vi "overlayfillcircle.vi"(0 "引用句柄输入":T1, 1 "数值":u8=25, 3 "Point1 (Pixels)":cluster{"X":sgl, "Y":sgl}, 5 "中心":cluster{"X":dbl, "Y":dbl}, 9 "偏移":cluster{"X":dbl, "Y":dbl}, 11 "错误输入（无错误）":errorcluster, 12 "分辨率":cluster{"X":sgl, "Y":sgl}={"X"=0.005, "Y"=0.005}, 14 "Point2 (Pixels)":cluster{"X":sgl, "Y":sgl}) -> (4 "引用句柄输出":T1, 10 "Point":cluster{"X":dbl, "Y":dbl}, 15 "错误输出":errorcluster)   [LabVIEW 2015]
uses:
  <vilib>/vision/Image Controls.llb/IMAQ Image.ctl
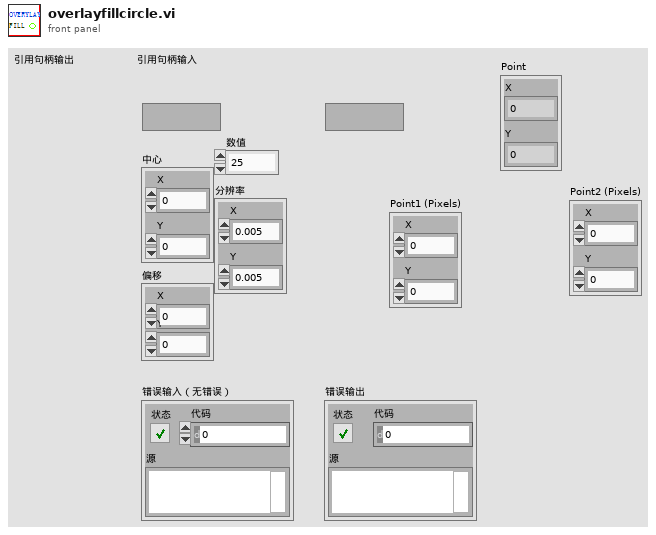
[diagram p1: front panel]
types:
  T1 = typedef "IMAQ Image.ctl" = refnum<image>
  T2 = cluster{"Left":i32, "Top":i32, "Right":i32, "Bottom":i32}
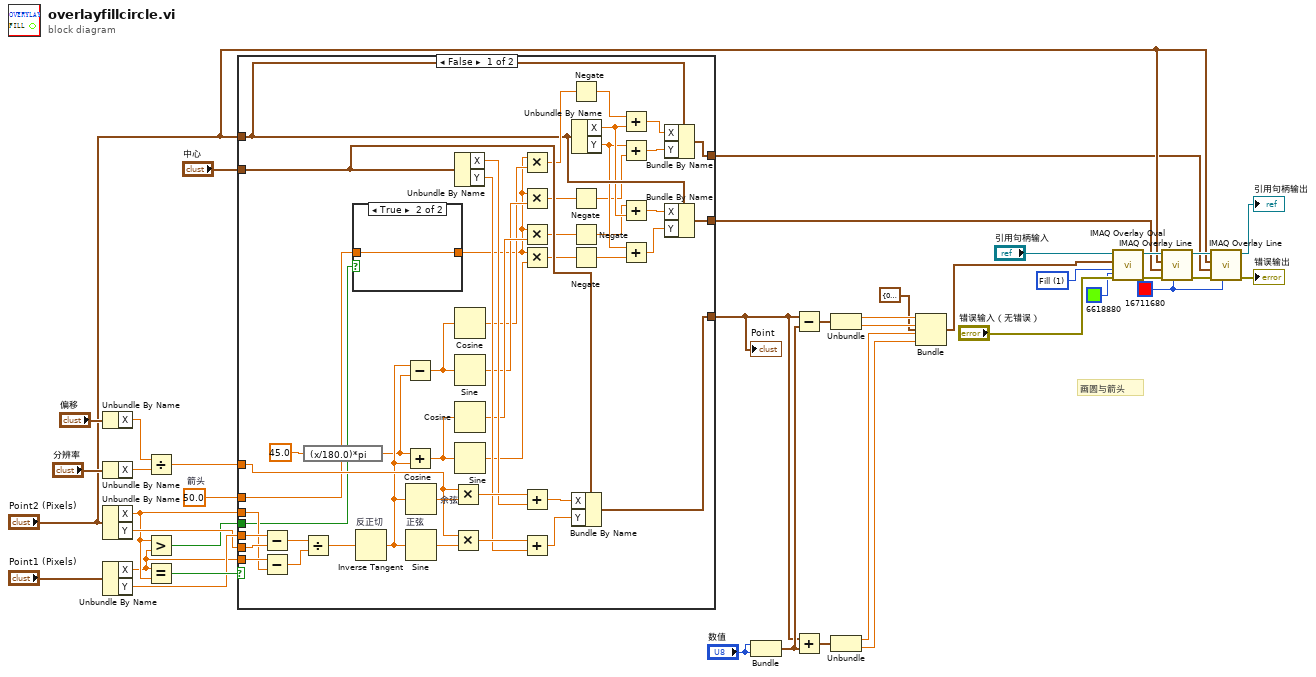
[diagram p0: block diagram]
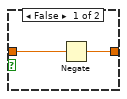
[diagram p2: hidden frame]
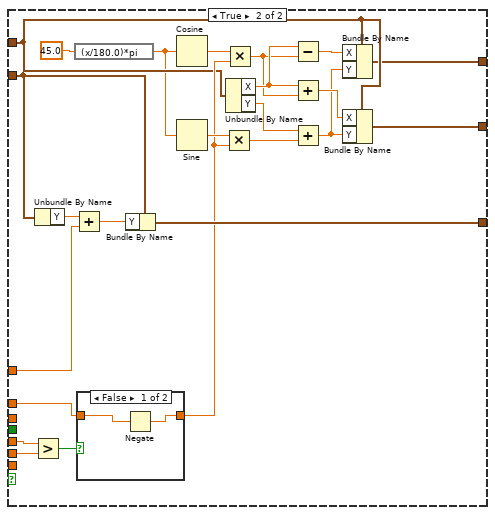
[diagram p3: hidden frame]
diagram:
  w1 = u32 16711680 ("Color")
  w5 = sgl 50.0  # 箭头
  w29 = u32 1 items=["Frame", "Fill"] ("Drawing Mode (Frame)")
  # "画圆与箭头"
  n1 = Unbundle By Name("偏移") -> ("X"=w22:dbl)
  n2 = Unbundle By Name("分辨率") -> ("X"=w20:sgl)
  n3 = Unbundle By Name("Point2 (Pixels)") -> ("X"=w8:sgl, "Y"=w16:sgl)
  n4 = Unbundle By Name("Point1 (Pixels)") -> ("X"=w7:sgl, "Y"=w17:sgl)
  n5 = Divide(x=w22, y=w20) -> (x/y=w18:dbl)
  n6 = Greater?(x=w8, y=w7) -> (0:w6:bool)
  n7 = Equal?(x=w7, y=w8) -> (x = y?=w24:bool)
  n8 = case shown="False" w24 {
    tunnel: "中心" -> [w77 w111]
    tunnel: w18 -> [w55 w113]
    tunnel: [w74 w112] -> w15
    tunnel: w17 -> [w86 w108]
    tunnel: w16 -> [w73 w107]
    tunnel: w7 -> [w46 _]
    tunnel: w8 -> [w45 _]
    tunnel: "Point2 (Pixels)" -> [w57 w98]
    tunnel: [w64 w99] -> w10
    tunnel: [w56 w97] -> w9
    tunnel: w6 -> [w44 _]
    tunnel: w5 -> [w40 w90]
    frame False {
      n9 = Subtract(x=w86, y=w73) -> (x-y=w85:sgl)
      n10 = Subtract(x=w46, y=w45) -> (x-y=w84:sgl)
      n11 = Divide(x=w85, y=w84) -> (x/y=w83:sgl)
      n12 = expression code="(x/180.0)*pi" ("degrees to radians")(45.0 ("Rotation")) -> (w41:dbl)
      n13 = case shown="True" w44 {
        tunnel: [w87 w89] -> w51
        tunnel: w40 -> [w88 w89]
        frame False {
          n14 = Negate(x=w88) -> (-x=w87:sgl)
        }
        frame True {
        }
      }
      n15 = Inverse Tangent "反正切"(1:w83) -> (0:w42:sgl)
      n16 = Subtract(x=w42, y=w41) -> (x-y=w63:dbl)
      n17 = Add(x=w41, y=w42) -> (x+y=w65:dbl)
      n18 = Cosine "余弦"(x=w42) -> (cos(x)=w72:sgl)
      n19 = Sine "正弦"(x=w42) -> (sin(x)=w82:sgl)
      n20 = Multiply(x=w55, y=w72) -> (x*y=w81:dbl)
      n21 = Multiply(x=w55, y=w82) -> (x*y=w79:dbl)
      n22 = Unbundle By Name(w77) -> ("X"=w80:dbl, "Y"=w78:dbl)
      n23 = Cosine(x=w63) -> (cos(x)=w58:dbl)
      n24 = Sine(x=w63) -> (sin(x)=w59:dbl)
      n25 = Cosine(x=w65) -> (cos(x)=w71:dbl)
      n26 = Sine(x=w65) -> (sin(x)=w70:dbl)
      n27 = Multiply(x=w51, y=w58) -> (x*y=w60:dbl)
      n28 = Multiply(x=w51, y=w59) -> (x*y=w61:dbl)
      n29 = Multiply(x=w51, y=w71) -> (x*y=w69:dbl)
      n30 = Multiply(x=w51, y=w70) -> (x*y=w68:dbl)
      n31 = Add(x=w81, y=w80) -> (x+y=w76:dbl)
      n32 = Add(x=w79, y=w78) -> (x+y=w75:dbl)
      n33 = Negate(x=w60) -> (-x=w47:dbl)
      n34 = Negate(x=w61) -> (-x=w48:dbl)
      n35 = Negate(x=w69) -> (-x=w49:dbl)
      n36 = Negate(x=w68) -> (-x=w50:dbl)
      n37 = Unbundle By Name(w57) -> ("X"=w54:sgl, "Y"=w53:sgl)
      n38 = Bundle By Name(cluster=w77, "X"=w76, "Y"=w75) -> (w74:cluster{"X":dbl, "Y":dbl})
      n39 = Add(x=w47, y=w54) -> (x+y=w62:dbl)
      n40 = Add(x=w53, y=w48) -> (x+y=w52:dbl)
      n41 = Add(x=w49, y=w54) -> (x+y=w66:dbl)
      n42 = Add(x=w53, y=w50) -> (x+y=w67:dbl)
      n43 = Bundle By Name(cluster=w57, "X"=w62, "Y"=w52) -> (w56:cluster{"X":sgl, "Y":sgl})
      n44 = Bundle By Name(cluster=w57, "X"=w66, "Y"=w67) -> (w64:cluster{"X":sgl, "Y":sgl})
    }
    frame True {
      n45 = Greater?(x=w108, y=w107) -> (0:w106:bool)
      n46 = Unbundle By Name(w111) -> ("Y"=w109:dbl)
      n47 = Add(x=w109, y=w113) -> (x+y=w110:dbl)
      n48 = expression code="(x/180.0)*pi" ("degrees to radians")(45.0 ("Rotation")) -> (w92:dbl)
      n49 = case shown="False" w106 {
        tunnel: [w114 w116] -> w103
        tunnel: w90 -> [w115 w116]
        frame False {
          n50 = Negate(x=w115) -> (-x=w114:sgl)
        }
        frame True {
        }
      }
      n51 = Bundle By Name(cluster=w111, "Y"=w110) -> (w112:cluster{"X":dbl, "Y":dbl})
      n52 = Cosine(x=w92) -> (cos(x)=w105:dbl)
      n53 = Sine(x=w92) -> (sin(x)=w104:dbl)
      n54 = Multiply(x=w104, y=w103) -> (x*y=w101:dbl)
      n55 = Multiply(x=w105, y=w103) -> (x*y=w95:dbl)
      n56 = Unbundle By Name(w98) -> ("X"=w96:sgl, "Y"=w102:sgl)
      n57 = Subtract(x=w96, y=w95) -> (x-y=w94:dbl)
      n58 = Add(x=w96, y=w95) -> (x+y=w100:dbl)
      n59 = Add(x=w102, y=w101) -> (x+y=w93:dbl)
      n60 = Bundle By Name(cluster=w98, "X"=w94, "Y"=w93) -> (w97:cluster{"X":sgl, "Y":sgl})
      n61 = Bundle By Name(cluster=w98, "X"=w100, "Y"=w93) -> (w99:cluster{"X":sgl, "Y":sgl})
    }
  }
  "Point" <- w15
  n62 = Bundle("数值"="数值", "数值"="数值") -> (w26:cluster{"数值":u8, "数值":u8})  [unwired: 1 in]
  n63 = Subtract(x=w15, y=w26) -> (x-y=w31:cluster{dbl, dbl})
  n64 = Add(x=w15, y=w26) -> (x+y=w34:cluster{dbl, dbl})
  n65 = Unbundle(w31) -> (w32:dbl, w33:dbl)
  n66 = Unbundle(w34) -> (w35:dbl, w36:dbl)
  n67 = Bundle(cluster=T2 {"Left"=0, "Top"=0, "Right"=0, "Bottom"=0} ("Bounding Rectangle"), "Left"=w32, "Top"=w33, "Right"=w35, "Bottom"=w36) -> (w37:T2)
  n68 = call "IMAQ Overlay Oval"("Color"=u32 6618880, "error in (no error)"="错误输入（无错误）", "Drawing Mode (Frame)"=w29, "Bounding Rectangle"=w37, "Image"="引用句柄输入") -> ("error out"=w4:errorcluster, "Image Out"=w14:T1)  [unwired: 5 in]
  n69 = call "IMAQ Overlay Line"("Color"=w1, "error in (no error)"=w4, "End Point"=w10, "Start Point"="Point2 (Pixels)", "Image"=w14) -> ("error out"=w3:errorcluster, "Image Out"=w13:T1)  [unwired: 5 in]
  n70 = call "IMAQ Overlay Line"("Color"=w1, "error in (no error)"=w3, "End Point"=w9, "Start Point"="Point2 (Pixels)", "Image"=w13) -> ("error out"=→"错误输出":errorcluster, "Image Out"=→"引用句柄输出":T1)  [unwired: 5 in]
